vi "ASI Enable Dark Subtract.vi"(10 "pcBMPPath":string, 11 "iCameraID":i32) -> (2 "pcBMPPath out":string, 3 "function return":i32)   [LabVIEW 2012, in "ASICamera2_no_err.lvlib"]
doc: "ASICAMERA_API ASI_ERROR_CODE ASIEnableDarkSubtract(int iCameraID, char *pcBMPPath);"
uses:
  <userlib>/ASICamera2_no_err/ASICamera2_no_err.lvlib
  <userlib>/ASICamera2_no_err/ASICamera2.dll
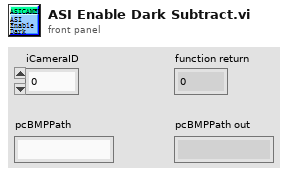
[diagram p1: front panel]
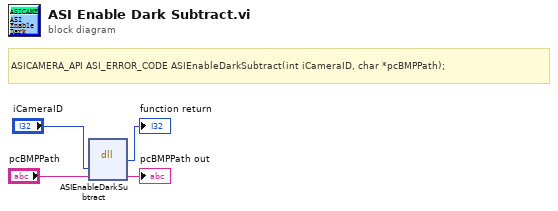
[diagram p0: block diagram]
diagram:
  # "ASICAMERA_API ASI_ERROR_CODE ASIEnableDarkSubtract(int iCameraID, char *pcBMPPath);"
  n1 = dll-call lib="D:/Program Files (x86)/National Instruments/LabVIEW 2012/user.lib/ASICamera2_no_err/ASICamera2.*" fn="ASIEnableDarkSubtract"("iCameraID"="iCameraID", "pcBMPPath"="pcBMPPath") -> (→"function return":i32, "pcBMPPath"=→"pcBMPPath out":string)  [unwired: 4 in, 2 out]
